vi "Normalise Vector.vi"(11 "Vector 3D":T1) -> (3 "Vector 3D Normalised":T1)   [LabVIEW 2022 SP3, in "3D.lvlib"]
uses:
  3D.lvlib
  Vector 3D.ctl
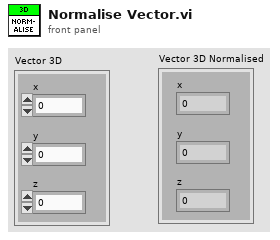
[diagram p1: front panel]
types:
  T1 = typedef "3D.lvlib/Vector 3D.ctl" = cluster{"x":sgl, "y":sgl, "z":sgl}
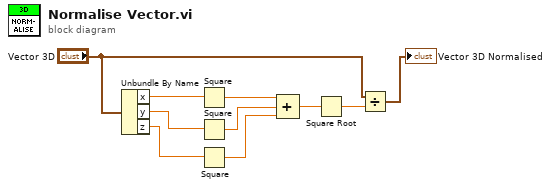
[diagram p0: block diagram]
diagram:
  n1 = Unbundle By Name("Vector 3D") -> ("x"=w10:sgl, "y"=w9:sgl, "z"=w8:sgl)
  n2 = Square(x=w10) -> (x^2=w7:sgl)
  n3 = Square(x=w9) -> (x^2=w6:sgl)
  n4 = Square(x=w8) -> (x^2=w5:sgl)
  n5 = Compound Arithmetic op=ADD(w7, w6, w5) -> (w4:sgl)
  n6 = Square Root(x=w4) -> (sqrt(x)=w2:sgl)
  n7 = Divide(x="Vector 3D", y=w2) -> (x/y=→"Vector 3D Normalised":T1)
